vi "Test_Observe_ViewModelPublication_OK.vi"(8 "error in (no error)":errorcluster, 11 "TestObservation In":refnum<class "TestObservation.lvclass">) -> (0 "error out":errorcluster, 3 "TestObservation Out":refnum<class "TestObservation.lvclass">)   [LabVIEW 2015, in "TestObservation.lvclass"]
uses:
  TestObservation.lvclass
  Framework/Mediator/Mediator/Mediator.lvclass
  PublishingViewModel/PublishingViewModel.lvclass
  Framework/IViewModel/IViewModel/IViewModel.lvclass/IViewModel.ctl
  Framework/IViewManager/IViewManager Messages/Launch Nested Views Msg/Launch Nested Views Msg.lvclass/Launch Nested Views Msg.ctl
  Framework/IViewManager/IViewManager/IViewManager.lvclass/IViewManager.ctl
  <vilib>/ActorFramework/Message Enqueuer/Message Enqueuer.lvclass/Message Enqueuer.ctl
  Framework/IViewManager/IViewManager Messages/Launch Nested Views Msg/Pack Launch Nested Views Msg.vi
  Framework/IViewManager/IViewManager/Write Startup Launch Nested Views Msg.vi
  <vilib>/ActorFramework/Message Enqueuer/Enqueue.vi
  <vilib>/ActorFramework/Message Priority Queue/Priority Enqueue.vi
  Framework/IViewable/IApplicationStyle/IApplicationStyle.lvclass
  Framework/IViewManager/IViewManager Messages/Launch Nested Views Msg/Launch Nested Views Msg.lvclass
  <vilib>/ActorFramework/Stop Msg/Stop Msg.lvclass
  <vilib>/addons/_JKI Toolkits/VI Tester/TestCase.llb/TestCase.lvclass
  Framework/IViewModel/IViewModel/IViewModel.lvclass
  <vilib>/ActorFramework/Actor/Actor.lvclass
  ObservingViewable/ObservingViewable.lvclass
  ObservingModel/ObservingModel.lvclass
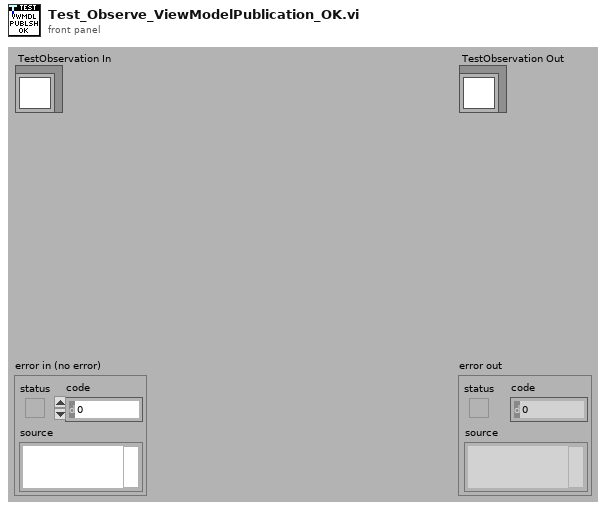
[diagram p1: front panel]
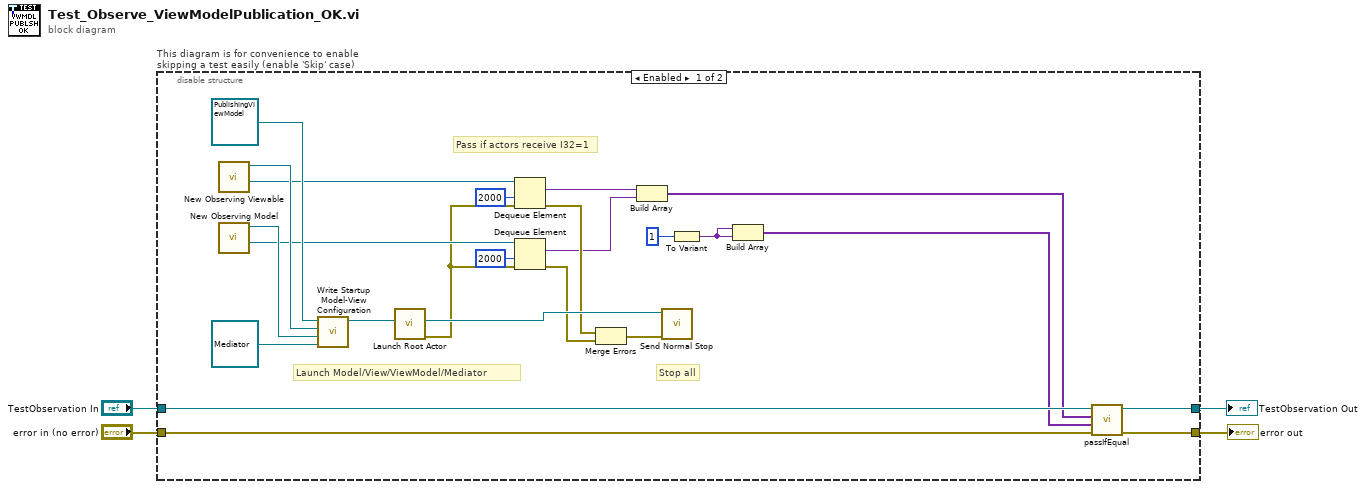
[diagram p0: block diagram]
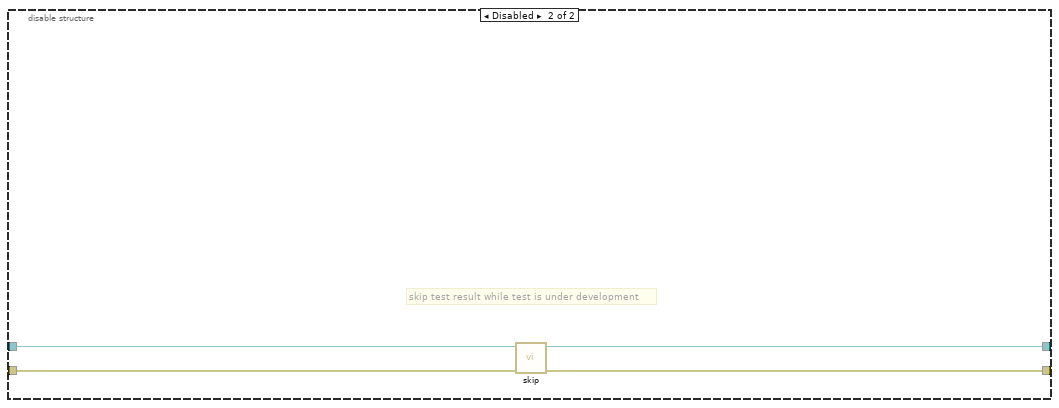
[diagram p2: hidden frame]
diagram:
  n1 = disable-structure "This diagram is for convenience to enable skipping a test easily (enable 'Skip' case)" shown="Enabled" {
    disable-tunnel: "TestObservation In" -> [w28 w32]
    disable-tunnel: [w27 w30] -> w1
    disable-tunnel: [w26 w31] -> w3
    disable-tunnel: "error in (no error)" -> [w25 w29]
    frame Enabled {
      # "Stop all"
      # "Launch Model/View/ViewModel/Mediator"
      # "Pass if actors receive I32=1"
      n2 = call "New Observing Viewable.vi"() -> ("Test Reply Queue"=w20:refnum<queue>, "ObservingViewable out"=w21:refnum<class "ObservingViewable.lvclass">)  [unwired: 10 in]
      n3 = call "New Observing Model.vi"() -> ("Test Reply Queue"=w13:refnum<queue>, "ObservingModel Out"=w15:refnum<class "ObservingModel.lvclass">)  [unwired: 10 in]
      n4 = call "Write Startup Model-View Configuration.vi"("Mediator Type"=refnum<class "Mediator.lvclass"> refnum ("Mediator.lvlib:Mediator.lvclass"), "Model Type"=w15, "Startup View Configuration"=w21, "IViewModel In"=refnum<class "PublishingViewModel.lvclass"> refnum ("PublishingViewModel.lvclass")) -> ("IViewModel Out"=w22:refnum<class "PublishingViewModel.lvclass">)  [unwired: 7 in]
      n5 = call <vilib>:"Launch Root Actor.vi"("Actor"=w22) -> ("error out"=w9:errorcluster, "Actor's Enqueuer"=w18:refnum<class "Message Enqueuer.lvclass">)  [unwired: 9 in]
      n6 = Dequeue Element(queue=w20, timeout in ms (-1)=2000, error in (no error)=w9) -> (element=w17:variant, error out=w10:errorcluster)  [unwired: 2 out]
      n7 = Dequeue Element(queue=w13, timeout in ms (-1)=2000, error in (no error)=w9) -> (element=w7:variant, error out=w12:errorcluster)  [unwired: 2 out]
      n8 = Merge Errors(w10, w12) -> (w11:errorcluster)
      n9 = Build Array(w17, w7) -> (w8:variant[])
      n10 = call <vilib>:"Send Normal Stop.vi"("error in (no error)"=w11, "Message Enqueuer"=w18) -> ()  [unwired: 9 in, 1 out]
      n11 = To Variant(anything=1) -> (Variant=w5:variant)
      n12 = Build Array(w5, w5) -> (w6:variant[])
      n13 = call-dynamic "passIfEqual.vi"("error in (no error)"=w25, "y"=w6, "x"=w8, "TestCase in"=w28) -> ("error out"=w26:errorcluster, "TestCase out"=w27:refnum<class "TestObservation.lvclass">)  [unwired: 6 in]
    }
    frame Disabled {
      # "skip test result while test is under development"
      n14 = call <vilib>:"skip.vi"("error in (no error)"=w29, "TestCase in"=w32) -> ("error out"=w31:errorcluster, "TestCase out"=w30:refnum<class "TestObservation.lvclass">)  [unwired: 8 in]
    }
  }
  "error out" <- w3
  "TestObservation Out" <- w1
